vi "FPGAmacroTDC.vi"() -> ()   [LabVIEW 2017]
uses:
  <vilib>/Platform/TimedLoop/XDataNode/timing_clust.ctl
  <vilib>/Platform/TimedLoop/XDataNode/nitl_modes.ctl
  <vilib>/Platform/TimedLoop/XDataNode/wakeup.ctl
  <vilib>/rvi/Emulation/niFpgaGetClockAttributes.vi
  <vilib>/rvi/Emulation/niFpgaSctlEmulationGetInTimedLoop.vi
  <vilib>/rvi/Emulation/niFpgaEmulationReportErrorSimple.vi
  <vilib>/rvi/Emulation/niFpgaProcessEmulError.vi
  <vilib>/rvi/eio/common/nirviEmuTemplateMethod_errors.vi
  <vilib>/rvi/Emulation/niFpgaCriticalErrorInLSC.vi
  <vilib>/rvi/Memory/Memory_Emulation/nirvimemoryEmulation.vi
  <vilib>/rvi/Memory/Memory_Emulation/nirvimemoryFastEmulation.vi
  <vilib>/rvi/DataTransferAndStorage/Container/Common/niFpgaContainerGetUniqueNameForEmu.vi
  <vilib>/rvi/Memory/Memory_Emulation/niFpgaMemoryEmulationCacheClearOnFirstRun.vi
  <vilib>/rvi/Memory/Memory_Emulation/nirvimemoryEmulationManagerCache_MakeExclusive.vi
  <vilib>/rvi/Memory/Memory_Emulation/niFpgaMemoryEmulationValidateCache.vi
  <vilib>/rvi/Memory/Memory_Emulation/nirvimemoryEmulationManagerCache_InsertValue.vi
  <vilib>/Utility/error.llb/Clear Errors.vi
  <vilib>/rvi/Memory/Memory_Emulation/nirvimemoryEmulationManagerCache_ReleaseExclusive.vi
  <vilib>/rvi/Memory/Memory_Emulation/nirvimemoryEmulationManagerCache_GetValue.vi
  <vilib>/rvi/Emulation/niFpgaEmulationIsFPGAContextNoSignature.vi
  <vilib>/rvi/Memory/Memory_Emulation/nirvimemoryEmulationManagerCache_SetValue.vi
  <vilib>/rvi/Emulation/niFpgaSctlEmulationResourceMgr.vi
  <vilib>/rvi/DataTransferAndStorage/Container/Common/niFpgaContainerExecOnDevCompGetState.vi
  <vilib>/rvi/errors/niFpgaSetErrorForExecOnDevCompSimple.vi
  <vilib>/rvi/eio/common/nirviEmuReportErrorAndStop.vi
  <vilib>/rvi/FIFO/Fifo_Resource/nirvififoEmulationSetSize.vi
  <vilib>/rvi/FIFO/Fifo_Resource/nirviFifoEmulationQueueMgr.vi
  <instcachedir>/0/nirviFifoEmulationQueueMgr_E5CAEC123FF24DC58D834DCA3CDAA9B5.lvgen/nirviFifoEmulationQueueMgr_E5CAEC123FF24DC58D834DCA3CDAA9B5_001.vi
  <vilib>/rvi/FIFO/Fifo_Resource/nirvififoEmulationDetermineInputValidOut.vi
  <vilib>/rvi/FIFO/Fifo_Resource/nirvififoEmulationCreateLock.vi
  <vilib>/rvi/FIFO/Fifo_Resource/nirvififoEmulationObtainLock.vi
  <vilib>/rvi/FIFO/Fifo_Resource/nirvififoEmulationReleaseLock.vi
  <vilib>/rvi/occurrence/nirviWaitOnOccurrenceBase.vi
  <vilib>/rvi/errors/nirviReportUnexpectedCaseInternalError.vi
  <vilib>/rvi/errors/nirviReportUnexpectedCaseInternalError (U32).vi
  <vilib>/rvi/interface/RandomDataEmulation/niFpgaRandomDataHandleErrors.vi
  <vilib>/rvi/DataTransferAndStorage/Container/Common/niFpgaContainerSetEmuInfo.vi
  <vilib>/eio/EIONode/EIONode.xnode
  <vilib>/Platform/TimedLoop/XDataNode/XDataNode.xnode
  <vilib>/rvi/DataTransferAndStorage/Container/XNode/niFpgaContainer.xnode
  <vilib>/rvi/FIFO/Fifo_Resource/niFpgaFifoEmulationRefIn.vi
  <vilib>/rvi/interface/RandomDataEmulation/nirviRandomDataFpgaReadWriteTemplate.vi
  <vilib>/addons/control/pid/fpga.llb/XNode/niFpgaPID.xnode
  <vilib>/rvi/LocalResourceManager/LocalResourceManager.xnode
  <vilib>/Platform/TimedLoop/XDataNode/XDNodeRunTimeDep.lvlib
panel:
  out "new data":bool=TRUE
  out "tau":u32
  in  "N photons":u32
  in  "Acquire times":bool
  in  "AO4 max":i16 min=0 max=3277
  in  "AO7":i16
  in  "AO6":i16
  in  "AO5":i16
  in  "D31":bool
  in  "D30":bool
  in  "D29":bool
  in  "D28":bool
  in  "D27":bool
  in  "D26":bool
  in  "D25":bool
  in  "D24":bool
  out "Seq DO bits":u64
  in  "High power":bool
  in  "Reinitialise controller":bool
  in  "PID gains":T1={"Proportional gain Kc"=0.0, "Integral time Ti [min]"=2.0, "Derivative time Td [min]"=0.0}
  in  "Controller output range":T2={"Output high"=10.0, "Output low"=-10.0}
  out "Control Signal 2":i16
  in  "Setpoint (L)":fxp<+/-,16,16> format="%.3f"
  out "Filtered Input":fxp<+/-,16,16>
  out "Filtered Input":i16(graph)
  out "Control Signal":i16(graph)
  out "Input Signal / mV":fxp<+/-,19,14> format="%.3g"
  out "Control Signal / mV":fxp<+/-,19,14> format="%.3g"
  in  "Setpoint (H)":fxp<+/-,16,16>
  in  "override noise eater?":bool
  in  "D23":bool
  in  "D22":bool
  in  "D21":bool
  in  "D20":bool
  in  "D19":bool
  in  "D18":bool
  in  "D17":bool
  in  "D16":bool
  in  "D15":bool
  in  "D14":bool
  in  "D13":bool
  in  "D12":bool
  out "coerced AO3 fl scan":i16
  in  "AO3 fl scan":i16
  out "Seq AO bits":u8
  in  "trigger data":u8
  in  "AO data":u8
  in  "time data":u32
  in  "count data":u8
  out "data waiting":bool
  in  "pulse number":u32
  in  "digout data":u64
  in  "Send photons?":bool
  out "Numeric":u32
  out "Array":u32[](array[numeric])
  in  "DIO11":bool
  in  "DIO5":bool
  in  "DIO4":bool
  in  "dds/ag":bool
  in  "AO1":bool
  in  "AO1 off":i16
  in  "AO1 on":i16
  in  "AO4":bool
  in  "AO4 off":i16
  in  "AO4 on":i16
  out "PMT COUNTS D":u32
  out "PMT COUNTS C":u32
  in  "AO3":bool
  in  "AO2":bool
  in  "AO3 off":i16
  in  "AO2 off":i16
  in  "AO3 on":i16
  in  "AO2 on":i16
  out "Error type":u8
  out "Error?":bool
  in  "Fl scan time":u32
  in  "Enum":enum16{"Pulse", "Fluorescence"}(ring)
  out "bin number":u32
  in  "ticks per bin":u32=40000000
  out "Frequency Chart":u32(graph)
  out "loop counter":u64
  in  "AOM":bool
  in  "DIO10":bool
  in  "Microwave":bool
  in  "EOM":bool
  in  "DIO6":bool
  in  "DIO7":bool
  in  "DIO9":bool
  in  "DIO8":bool
  out "PMT saturation":bool
  out "Slave loop selector":u8
  in  "AO7":i16
  in  "AO6":i16
  in  "start sequence":bool
  in  "Line trig?":bool
  in  "# of pulses":i32
  in  "Debug counts?":bool
  in  "# of runs":i32
  out "Fifo Timed Out (B)":bool
  out "PMT COUNTS A":u32
  out "Fifo Timed Out (A)":bool
  out "PMT COUNTS B":u32
  # "Seb AO"
  # "Scan type:"
  # "Load AO memory"
  # "Fluorescence scan"
  # "Pulse sequencer"
  # "Globals"
  # "369 drift lock"
  # "List of error types:\n\n1: AO3 (AOM) voltage out of range."
  # "Crud:"
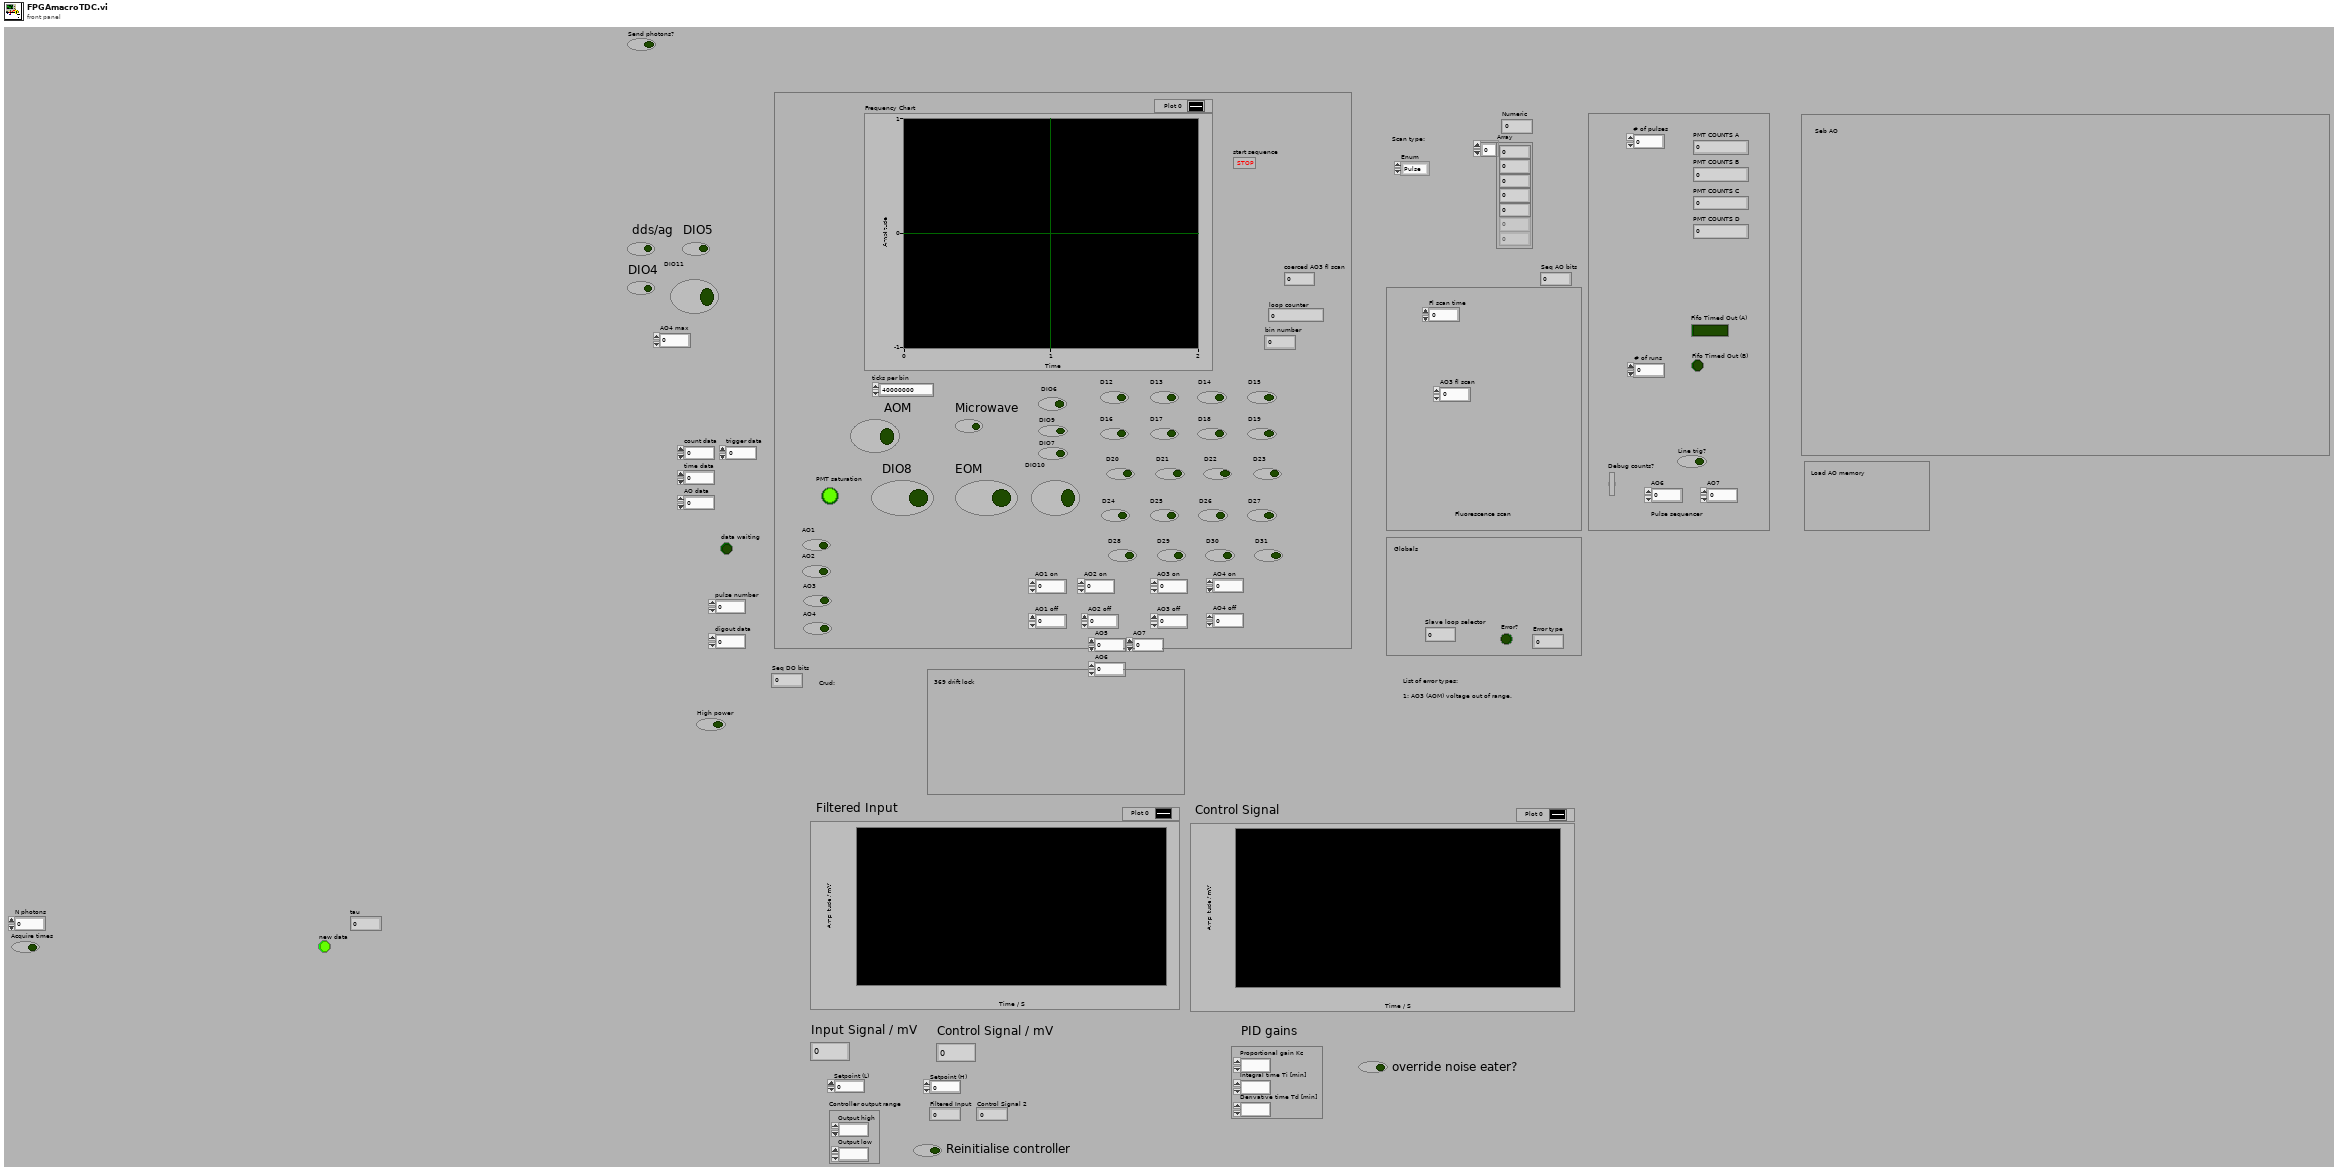
[diagram p1: front panel]
types:
  T1 = cluster{"Proportional gain Kc":fxp<+/-,16,8>, "Integral time Ti [min]":fxp<+/-,16,8>, "Derivative time Td [min]":fxp<+/-,16,8>}
  T2 = cluster{"Output high":fxp<+/-,16,16>, "Output low":fxp<+/-,16,16>}
  T3 = typedef "XDNodeRunTimeDep.lvlib/timing_clust.ctl" = cluster{"Expected End [f-1]":u64, "Actual End [f-1]":u64, "Finished Late? [f-1]":bool, "Expected End [i-1]":u64, "Actual End [i-1]":u64, "Finished Late? [i-1]":bool, "Expected Start [i]":u64, "Actual Start [i]":u64, "Expected Start [f]":u64, "Actual Start [f]":u64, "Source Name":string, "Structure Name":string, "Period":i64, "Deadline":i64, "Offset":i64, "Start":i64, "Priority":i32, "Timeout":i32, "Mode":T4, "Wakeup Reason":T5, "Error":errorcluster, "Source Type":string, "Secondary Source Type":string, "Global End Time":u64, "Global Start Time":u64, "Frame Duration":u64, "Iteration Duration":u64, "Assigned CPU":i32, "I/O Scan Engine Mode":u32}
  T4 = typedef "XDNodeRunTimeDep.lvlib/nitl_modes.ctl" = enum32{"No Change", "Process missed periods, maintain original phase", "Discard missed periods, maintain original phase", "Process missed periods, ignore original phase", "Discard missed periods, ignore original phase"}
  T5 = typedef "XDNodeRunTimeDep.lvlib/wakeup.ctl" = enum32{"Normal", "Aborted", "Asynchronous wakeup", "Timing source error", "Timed loop error", "Timeout"}
  T6 = cluster{"Boolean array[0]":bool, "Boolean array[1]":bool, "Boolean array[2]":bool, "Boolean array[3]":bool}
  T7 = cluster{"proportional gain (Kc)":i16, "integral gain (Kc*Ts/Ti)":i16, "derivative gain (Kc*Td/Ts)":i16}
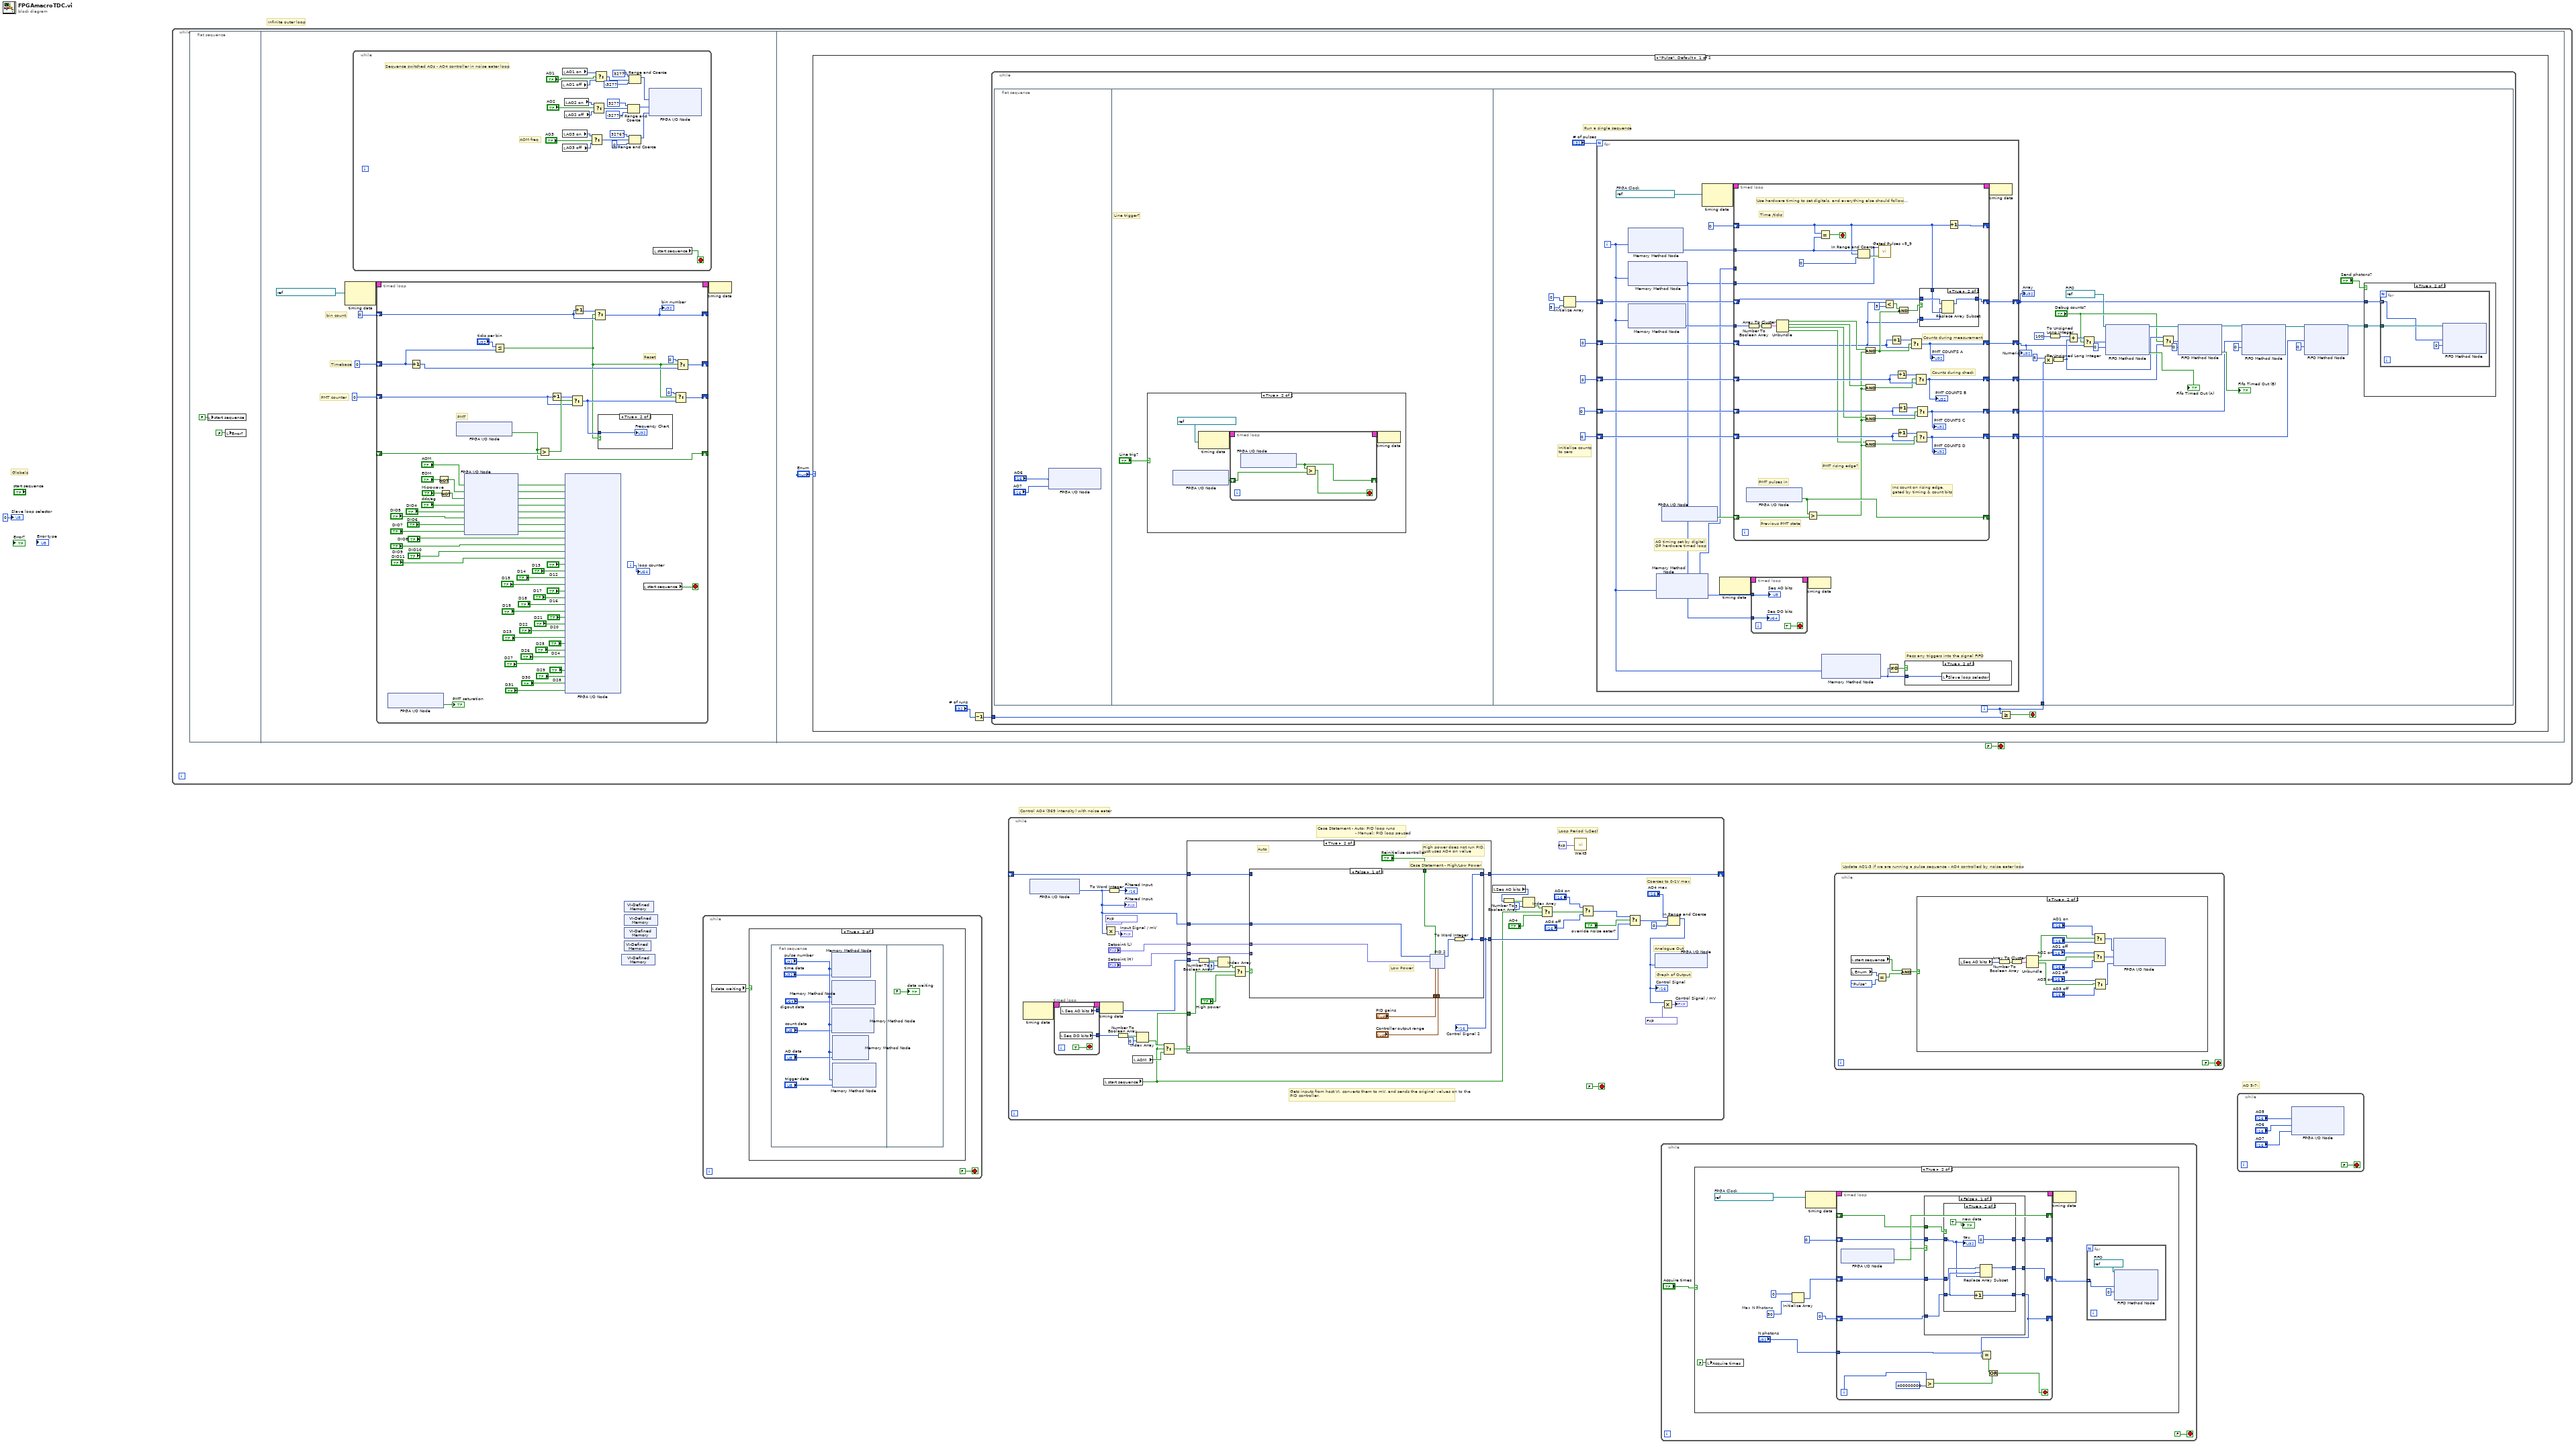
[diagram p0: block diagram]
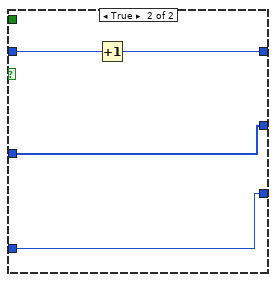
[diagram p4: hidden frame]
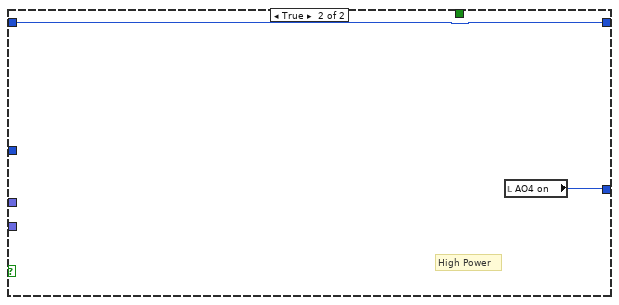
[diagram p6: hidden frame]
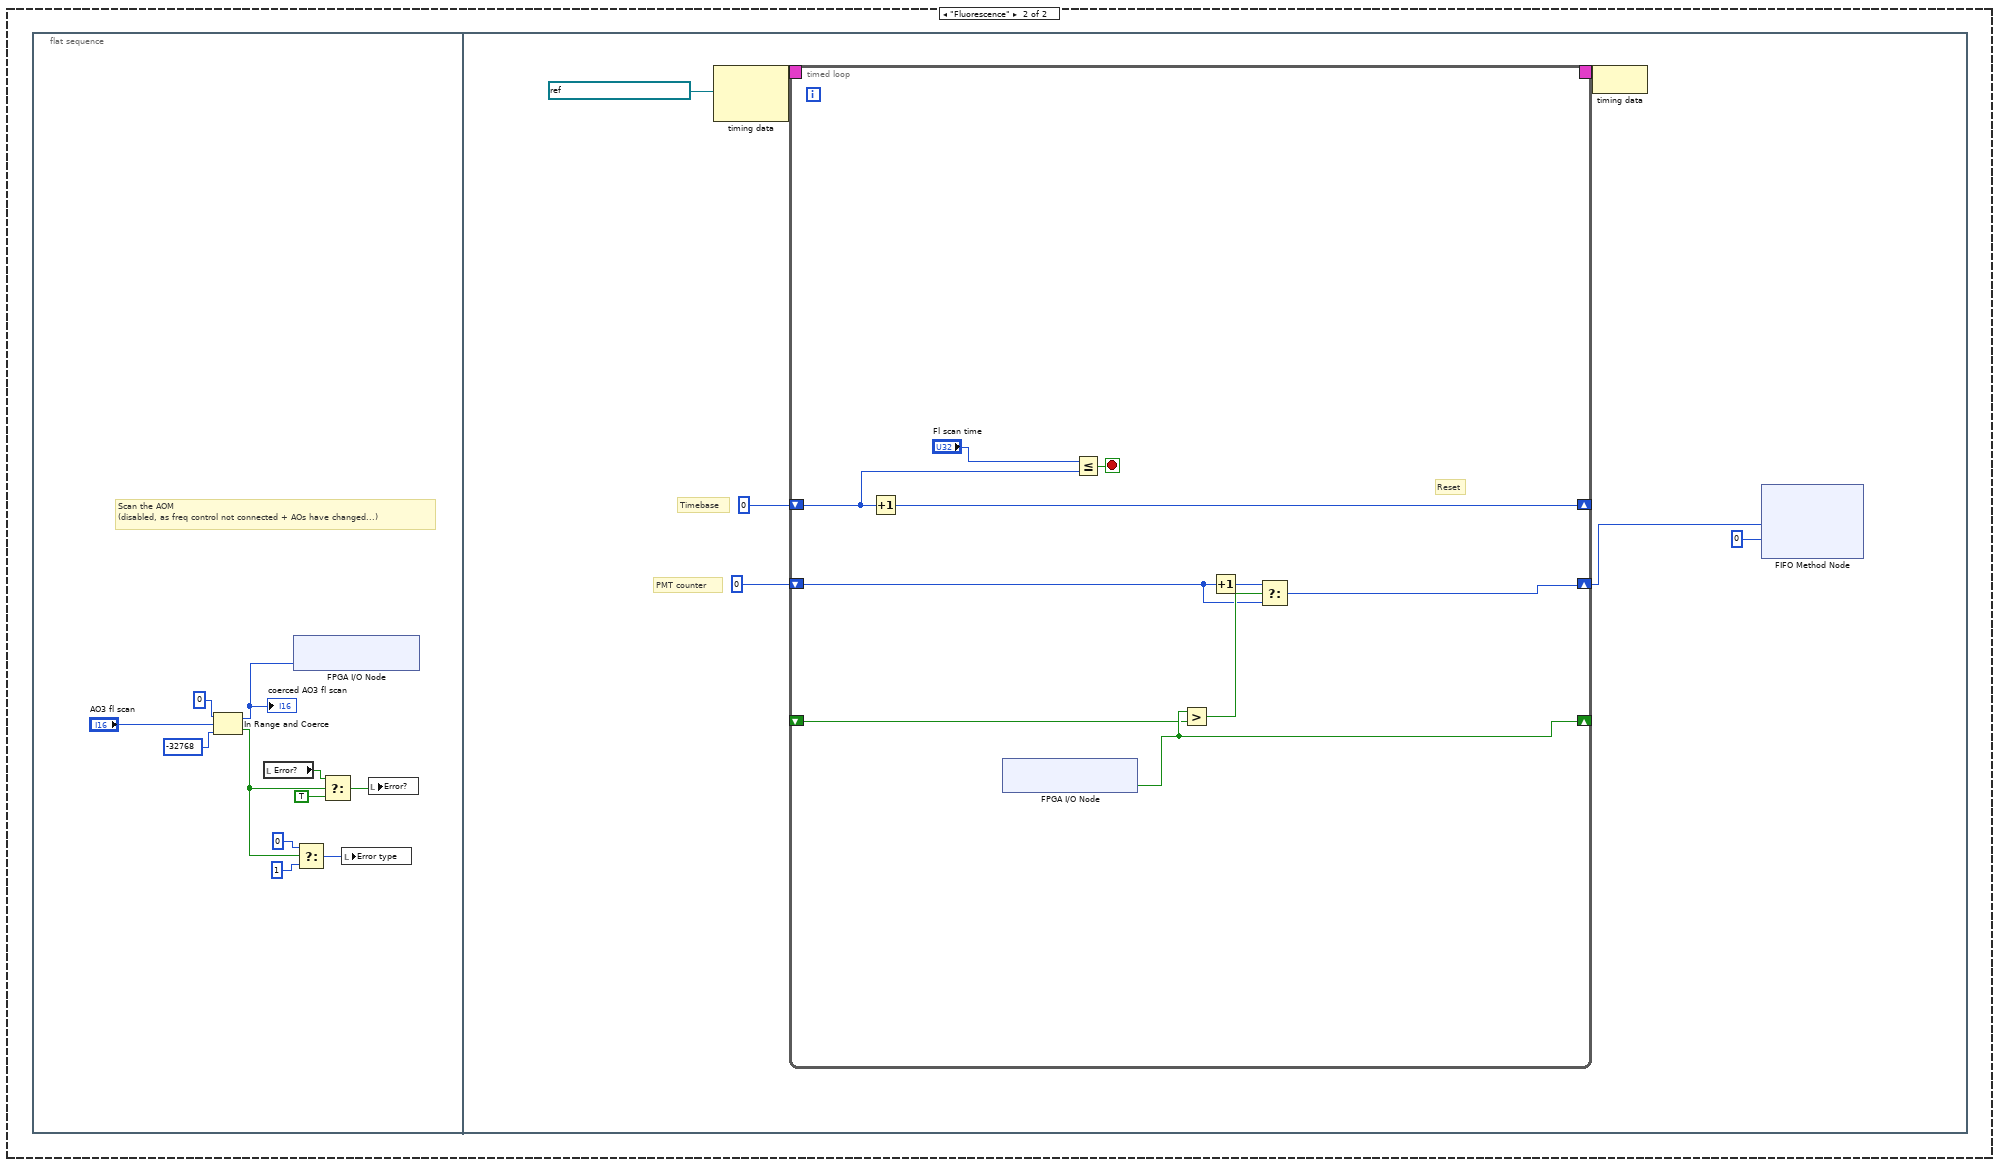
[diagram p14: hidden frame]
diagram:
  # "Control AO4 (369 intensity) with noise eater"
  # "Update AO1-3 if we are running a pulse sequence - AO4 controlled by noise eater loop"
  # "AO 5-7:"
  # "Globals"
  # "Infinite outer loop"
  n1 = while {
    stop <- FALSE stop-if-true
    n2 = flat-sequence {
      frame #0 {
        n3 = local write "start sequence"(FALSE ("start sequence")) -> ()
        n4 = local write "Error?"(FALSE ("Error?")) -> ()
      }
      frame #1 {
        # "bin count"
        # "PMT counter"
        # "Timebase"
        n5 = node-c288(refnum<k21> "40 MHz Onboard Clock" ("FPGA Clock To Enable")) -> (w10:T3)  [unwired: 1 in]
        n6 = while {
          stop <- w93 stop-if-true
          # "AOM freq"
          # "Sequence switched AOs - AO4 controller in noise eater loop"
          n7 = local read "AO1 off"() -> (w75:i16)
          n8 = local read "AO1 on"() -> (w76:i16)
          n9 = local read "AO3 on"() -> (w86:i16)
          n10 = local read "AO3 off"() -> (w85:i16)
          n11 = local read "AO2 on"() -> (w88:i16)
          n12 = local read "AO2 off"() -> (w87:i16)
          n13 = Select(t=w86, s="AO3", f=w85) -> (s? t:f=w82:i16)
          n14 = Select(t=w88, s="AO2", f=w87) -> (s? t:f=w81:i16)
          n15 = Select(t=w76, s="AO1", f=w75) -> (s? t:f=w77:i16)
          n16 = In Range and Coerce(upper limit=i16 3277, x=w81, lower limit=i16 -3277) -> (coerced(x)=w92:i16)  [unwired: 1 out]
          n17 = In Range and Coerce(upper limit=i16 32767, x=w82, lower limit=i16 0) -> (coerced(x)=w89:i16)  [unwired: 1 out]
          n18 = In Range and Coerce(upper limit=i16 3277, x=w77, lower limit=i16 -3277) -> (coerced(x)=w78:i16)  [unwired: 1 out]
          n19 = xnode "FPGA I/O Node"("Connector0/AO1"=w78, "Connector0/AO2"=w92, "Connector0/AO3"=w89) -> ()  [unwired: 3 in, 3 out]
          n20 = local read "start sequence"() -> (w93:bool)
        }
        n21 = timed-loop {
          timing: w10 -> [_]
          timing-out: [_] -> w9
          shift-right: [w62] -> _
          shift-left: u32 0 -> [w55]
          shift-right: [w60] -> _
          shift-left: u32 0 -> [w57]
          shift-right: [w45] -> _
          shift-left: _ -> [w53]
          shift-right: [w49] -> _
          shift-left: u32 0 -> [w47]
          i -> [w54]
          stop <- w50 stop-if-true
          # "PMT"
          # "Reset"
          n22 = xnode "FPGA I/O Node"() -> ("Connector0/DIO13"=→"PMT saturation":bool)  [unwired: 1 in, 1 out]
          n23 = Increment(x=w55) -> (x+1=w64:u32)
          n24 = Not(x="EOM") -> (.not. x?=w12:bool)
          n25 = Not(x="Microwave") -> (.not. x?=w43:bool)
          n26 = xnode "FPGA I/O Node"() -> ("Connector0/DIO15"=w45:bool)  [unwired: 1 in, 1 out]
          n27 = xnode "FPGA I/O Node"("Connector0/DIO0"="AOM", "Connector0/DIO1"=w12, "Connector0/DIO2"=w43, "Connector0/DIO3"="dds/ag", "Connector0/DIO4"="DIO4", "Connector0/DIO5"="DIO5", "Connector0/DIO6"="DIO6", "Connector0/DIO7"="DIO7") -> ()  [unwired: 8 in, 8 out]
          n28 = Less Or Equal?(x="ticks per bin", y=w55) -> (x <= y?=w46:bool)
          n29 = Greater?(x=w45, y=w53) -> (0:w58:bool)
          n30 = Increment(x=w57) -> (x+1=w61:u32)
          n31 = xnode "FPGA I/O Node"("Connector1/DIO0"="AOM", "Connector1/DIO1"=w12, "Connector1/DIO2"=w43, "Connector1/DIO3"="dds/ag", "Connector1/DIO4"="DIO4", "Connector1/DIO5"="DIO5", "Connector1/DIO6"="DIO6", "Connector1/DIO7"="DIO7", "Connector1/DIO8"="DIO8", "Connector1/DIO9"="DIO9", "Connector1/DIO10"="DIO10", "Connector1/DIO11"="DIO11", "Connector1/DIO12"="D12", "Connector1/DIO13"="D13", "Connector1/DIO14"="D14", "Connector1/DIO15"="D15", "Connector1/DIO16"="D16", "Connector1/DIO17"="D17", "Connector1/DIO18"="D18", "Connector1/DIO19"="D19", "Connector1/DIO20"="D20", "Connector1/DIO21"="D21", "Connector1/DIO22"="D22", "Connector1/DIO23"="D23", "Connector1/DIO24"="D24", "Connector1/DIO25"="D25", "Connector1/DIO26"="D26", "Connector1/DIO27"="D27", "Connector1/DIO28"="D28", "Connector1/DIO29"="D29", "Connector1/DIO30"="D30", "Connector1/DIO31"="D31") -> ()  [unwired: 32 in, 32 out]
          n32 = Select(t=w61, s=w58, f=w57) -> (s? t:f=w51:u32)
          n33 = Increment(x=w47) -> (x+1=w48:u32)
          n34 = Select(t=w48, s=w46, f=w47) -> (s? t:f=w49:u32)
          "bin number" <- w49
          n35 = case shown="True" w46 {
            tunnel: w51 -> [_ w65]
            frame False {
            }
            frame True {
              "Frequency Chart" <- w65
            }
          }
          n36 = local read "start sequence"() -> (w50:bool)
          n37 = Select(t=u32 0, s=w46, f=w51) -> (s? t:f=w60:u32)
          n38 = Select(t=u32 0, s=w46, f=w64) -> (s? t:f=w62:u32)
          "loop counter" <- w54
        }
        n39 = node-c288(w9) -> ()
      }
      frame #2 {
        n40 = case shown="\"Pulse\", Default" "Enum" {
          frame "Pulse", Default {
            n41 = Decrement(x="# of runs") -> (x-1=w95:i32)
            n42 = while {
              tunnel: w95 -> [w98]
              i -> [w99]
              stop <- w97 stop-if-true
              n43 = flat-sequence {
                tunnel: w99 -> [w131]
                frame #0 {
                  n44 = xnode "FPGA I/O Node"("Connector0/AO6"="AO6", "Connector0/AO7"="AO7") -> ()  [unwired: 2 in, 2 out]
                }
                frame #1 {
                  # "Line trigger?"
                  n45 = case shown="True" "Line trig?" {
                    frame False {
                    }
                    frame True {
                      n46 = xnode "FPGA I/O Node"() -> ("Connector0/DIO14"=w103:bool)  [unwired: 1 in, 1 out]
                      n47 = node-c288(refnum<k21> "40 MHz Onboard Clock" ("Source Name")) -> (w106:T3)
                      n48 = timed-loop {
                        timing: w106 -> [_]
                        timing-out: [_] -> w105
                        shift-right: [w108] -> _
                        shift-left: w103 -> [w109]
                        stop <- w107 stop-if-true
                        n49 = xnode "FPGA I/O Node"() -> ("Connector0/DIO14"=w108:bool)  [unwired: 1 in, 1 out]
                        n50 = Greater?(x=w108, y=w109) -> (0:w107:bool)
                      }
                      n51 = node-c288(w105) -> ()
                    }
                  }
                }
                frame #2 {
                  w119 = refnum<k21> "U32 FIFO"  # FIFO
                  # "Run a single sequence"
                  # "Initialize counts\nto zero"
                  n52 = Initialize Array(u32 0 ("element"), 5 ("dimension size")) -> (w120:u32[])
                  n53 = for {
                    N: "# of pulses" -> [_]
                    shift-right: [w176] -> w137
                    shift-left: u32 0 -> [w174]
                    shift-right: [w175] -> w139
                    shift-left: u32 0 -> [w173]
                    shift-right: [w168] -> w124
                    shift-left: u32 0 -> [w169]
                    shift-right: [w166] -> w123
                    shift-left: u32 0 -> [w167]
                    shift-right: [w164] -> w116
                    shift-left: w120 -> [w165]
                    i -> [w161]
                    w177 = refnum<k21> "40 MHz Onboard Clock"  # FPGA Clock
                    # "AO timing set by digital\nOP hardware timed loop"
                    # "Pass any triggers into the signal FIFO"
                    n54 = xnode ("Memory Method Node")("Address"=w161) -> ("Data"=w158:u64)  [unwired: 1 in, 1 out]
                    n55 = xnode ("Memory Method Node")("Address"=w161) -> ("Data"=w163:u32)  [unwired: 1 in, 1 out]
                    n56 = xnode ("Memory Method Node")("Address"=w161) -> ("Data"=w162:u8)  [unwired: 1 in, 1 out]
                    n57 = xnode ("Memory Method Node")("Address"=w161) -> ("Data"=w160:u8)  [unwired: 1 in, 1 out]
                    n58 = xnode "FPGA I/O Node"() -> ("Connector0/DIO15"=w171:bool)  [unwired: 1 in, 1 out]
                    n59 = node-c288(w177) -> (w179:T3)  [unwired: 1 in]
                    n60 = node-c288() -> (w157:T3)  [unwired: 1 in]
                    n61 = timed-loop {
                      timing: w179 -> [_]
                      timing-out: [_] -> w178
                      shift-right: [w219] -> w176
                      shift-left: w174 -> [w189]
                      shift-right: [w225] -> _
                      shift-left: w171 -> [w224]
                      shift-right: [w209] -> _
                      shift-left: u32 0 -> [w188]
                      shift-right: [w217] -> w175
                      shift-left: w173 -> [w221]
                      tunnel: w158 -> [w211]
                      tunnel: w162 -> [w210]
                      tunnel: w163 -> [w208]
                      shift-right: [w202] -> w168
                      shift-left: w169 -> [w204]
                      shift-right: [w198] -> w166
                      shift-left: w167 -> [w199]
                      shift-right: [w190] -> w164
                      shift-left: w165 -> [w192]
                      tunnel: w160 -> [_]
                      stop <- w218 stop-if-true
                      # "Use hardware timing to set digitals, and everything else should follow..."
                      # "Previous PMT state"
                      # "Counts during check"
                      # "Counts during measurement"
                      # "Time /ticks"
                      # "Inc count on rising edge,\ngated by timing & count bits"
                      # "PMT rising edge?"
                      # "PMT pulses in"
                      n62 = xnode "FPGA I/O Node"() -> ("Connector0/DIO15"=w225:bool)  [unwired: 1 in, 1 out]
                      n63 = Number To Boolean Array(number=w210) -> (Boolean array=w214:bool[])
                      n64 = Array To Cluster(array=w214) -> (cluster=w213:T6)
                      n65 = Unbundle(w213) -> ("Boolean array[0]"=w207:bool, "Boolean array[1]"=w212:bool, "Boolean array[2]"=w203:bool, "Boolean array[3]"=w196:bool)
                      n66 = Greater?(x=w225, y=w224) -> (0:w197:bool)
                      n67 = Equal?(x=w188, y=w208) -> (x = y?=w218:bool)
                      n68 = In Range and Coerce(upper limit=w208, x=w188, lower limit=u32 0) -> (In Range?=w216:bool)  [unwired: 1 out]
                      n69 = And(x=w207, y=w197) -> (x .and. y?=w193:bool)
                      n70 = And(x=w212, y=w197) -> (x .and. y?=w220:bool)
                      n71 = And(x=w203, y=w197) -> (x .and. y?=w205:bool)
                      n72 = And(x=w196, y=w197) -> (x .and. y?=w200:bool)
                      n73 = call "Gated Pulses v5_9.vi"("Gate"=w216, "Pulse bits"=w211) -> ()  [unwired: 3 in]
                      n74 = Less?(x=w189, y=i16 5) -> (x < y?=w194:bool)
                      n75 = Increment(x=w189) -> (x+1=w223:u32)
                      n76 = Increment(x=w221) -> (x+1=w222:u32)
                      n77 = Increment(x=w199) -> (x+1=w201:u32)
                      n78 = Increment(x=w204) -> (x+1=w206:u32)
                      n79 = And(x=w194, y=w193) -> (x .and. y?=w191:bool)
                      n80 = Select(t=w223, s=w193, f=w189) -> (s? t:f=w219:u32)
                      "PMT COUNTS A" <- w219
                      n81 = Select(t=w222, s=w220, f=w221) -> (s? t:f=w217:u32)
                      "PMT COUNTS B" <- w217
                      n82 = Select(t=w201, s=w200, f=w199) -> (s? t:f=w198:u32)
                      "PMT COUNTS D" <- w198
                      n83 = Select(t=w206, s=w205, f=w204) -> (s? t:f=w202:u32)
                      "PMT COUNTS C" <- w202
                      n84 = case shown="True" w191 {
                        tunnel: w192 -> [w226 w230]
                        tunnel: [w226 w229] -> w190
                        tunnel: w189 -> [_ w227]
                        tunnel: w188 -> [_ w228]
                        frame False {
                        }
                        frame True {
                          n85 = Replace Array Subset(array=w230, new element=w228, index=w227) -> (w229:u32[])
                        }
                      }
                      n86 = Increment(x=w188) -> (x+1=w209:u32)
                    }
                    n87 = timed-loop {
                      timing: w157 -> [_]
                      timing-out: [_] -> w156
                      tunnel: w160 -> [w182]
                      tunnel: w158 -> [w181]
                      stop <- TRUE stop-if-true
                      "Seq AO bits" <- w182
                      "Seq DO bits" <- w181
                    }
                    n88 = node-c288(w156) -> ()
                    n89 = xnode ("Memory Method Node")("Address"=w161) -> ("Data"=w159:u8)  [unwired: 1 in, 1 out]
                    n90 = Not Equal To 0?(x=w159) -> (x != 0?=w170:bool)
                    n91 = case shown="True" w170 {
                      tunnel: w159 -> [_ w187]
                      frame False {
                      }
                      frame True {
                        n92 = local write "Slave loop selector"(w187) -> ()
                      }
                    }
                    n93 = node-c288(w178) -> ()
                  }
                  "Array" <- w116
                  "Numeric" <- w137
                  n94 = Multiply(x=5 ("y"), y=w131) -> (x*y=w144:i32)
                  n95 = To Unsigned Long Integer(number=i16 100) -> (unsigned 32bit integer=w145:u32)
                  n96 = To Unsigned Long Integer(number=w144) -> (unsigned 32bit integer=w143:u32)
                  n97 = Add(x=w145, y=w143) -> (x+y=w141:u32)
                  n98 = Select(t=w141, s="Debug counts?", f=w137) -> (s? t:f=w140:u32)
                  n99 = xnode ("FIFO Method Node")("Element"=w140, "Timeout"=0, "FIFO In"=w119) -> ("Timed Out?"=→"Fifo Timed Out (A)":bool, "FIFO Out"=w148:refnum<k21>)
                  n100 = Select(t=w143, s="Debug counts?", f=w139) -> (s? t:f=w142:u32)
                  n101 = xnode ("FIFO Method Node")("Element"=w142, "Timeout"=0, "FIFO In"=w148) -> ("Timed Out?"=→"Fifo Timed Out (B)":bool, "FIFO Out"=w128:refnum<k21>)
                  n102 = xnode ("FIFO Method Node")("Element"=w124, "Timeout"=0, "FIFO In"=w128) -> ("FIFO Out"=w127:refnum<k21>)  [unwired: 1 out]
                  n103 = xnode ("FIFO Method Node")("Element"=w123, "Timeout"=0, "FIFO In"=w127) -> ("FIFO Out"=w117:refnum<k21>)  [unwired: 1 out]
                  n104 = case shown="True" "Send photons?" {
                    tunnel: w117 -> [_ w152]
                    tunnel: w116 -> [_ w151]
                    frame False {
                    }
                    frame True {
                      n105 = for {
                        tunnel: w152 -> [w155]
                        tunnel: w151 -> [w153] mode=indexing
                        n106 = xnode ("FIFO Method Node")("Element"=w153, "Timeout"=0, "FIFO In"=w155) -> ()  [unwired: 2 out]
                      }
                    }
                  }
                }
              }
              n107 = Greater Or Equal?(x=w99, y=w98) -> (x >= y?=w97:bool)
            }
          }
          frame "Fluorescence" {
            n108 = flat-sequence {
              frame #0 {
                # "Scan the AOM\n(disabled, as freq control not connected + AOs have changed...)"
                n109 = In Range and Coerce(upper limit=i16 0, x="AO3 fl scan", lower limit=i16 -32768) -> (coerced(x)=w245:i16, In Range?=w240:bool)
                "coerced AO3 fl scan" <- w245
                n110 = local read "Error?"() -> (w244:bool)
                n111 = xnode "FPGA I/O Node"("Connector0/AO3"=w245) -> ()  [unwired: 1 in, 1 out]
                n112 = Select(t=u8 0, s=w240, f=u8 1) -> (s? t:f=w241:u8)
                n113 = Select(t=w244, s=w240, f=TRUE) -> (s? t:f=w242:bool)
                n114 = local write "Error type"(w241) -> ()
                n115 = local write "Error?"(w242) -> ()
              }
              frame #1 {
                # "PMT counter"
                # "Timebase"
                n116 = node-c288(refnum<k21> "40 MHz Onboard Clock" ("FPGA Clock To Enable")) -> (w254:T3)  [unwired: 1 in]
                n117 = timed-loop {
                  timing: w254 -> [_]
                  timing-out: [_] -> w253
                  shift-right: [w255] -> _
                  shift-left: u32 0 -> [w261]
                  shift-right: [w257] -> w248
                  shift-left: u32 0 -> [w262]
                  shift-right: [w260] -> _
                  shift-left: _ -> [w259]
                  stop <- w256 stop-if-true
                  # "Reset"
                  n118 = Increment(x=w261) -> (x+1=w255:u32)
                  n119 = xnode "FPGA I/O Node"() -> ("Connector0/DIO15"=w260:bool)  [unwired: 1 in, 1 out]
                  n120 = Less Or Equal?(x="Fl scan time", y=w261) -> (x <= y?=w256:bool)
                  n121 = Greater?(x=w260, y=w259) -> (0:w263:bool)
                  n122 = Increment(x=w262) -> (x+1=w264:u32)
                  n123 = Select(t=w264, s=w263, f=w262) -> (s? t:f=w257:u32)
                }
                n124 = node-c288(w253) -> ()
                n125 = xnode ("FIFO Method Node")("Element"=w248, "Timeout"=0) -> ()  [unwired: 1 in, 2 out]
              }
            }
          }
        }
      }
    }
  }
  n126 = xnode "VI-Defined Memory"() -> ()  [unwired: 1 out]
  n127 = xnode "VI-Defined Memory"() -> ()  [unwired: 1 out]
  n128 = xnode "VI-Defined Memory"() -> ()  [unwired: 1 out]
  n129 = xnode "VI-Defined Memory"() -> ()  [unwired: 1 out]
  n130 = xnode "VI-Defined Memory"() -> ()  [unwired: 1 out]
  n131 = while {
    stop <- FALSE stop-if-true
    n132 = local read "data waiting"() -> (w272:bool)
    n133 = case shown="True" w272 {
      frame False {
      }
      frame True {
        n134 = flat-sequence {
          frame #0 {
            n135 = xnode ("Memory Method Node")("Address"="pulse number", "Data"="time data") -> ()  [unwired: 1 in, 1 out]
            n136 = xnode ("Memory Method Node")("Address"="pulse number", "Data"="digout data") -> ()  [unwired: 1 in, 1 out]
            n137 = xnode ("Memory Method Node")("Address"="pulse number", "Data"="count data") -> ()  [unwired: 1 in, 1 out]
            n138 = xnode ("Memory Method Node")("Address"="pulse number", "Data"="AO data") -> ()  [unwired: 1 in, 1 out]
            n139 = xnode ("Memory Method Node")("Address"="pulse number", "Data"="trigger data") -> ()  [unwired: 1 in, 1 out]
          }
          frame #1 {
            "data waiting" <- FALSE
          }
        }
      }
    }
  }
  n140 = while {
    shift-right: [w292] -> _
    shift-left: _ -> [w291]
    stop <- FALSE stop-if-true
    # "Coerces to 0-1V max"
    # "Graph of Output"
    # "Gets inputs from host VI, converts them to mV, and sends the original values on to the PID controller."
    # "Case Statement - Auto: PID loop runs\n                            - Manual: PID loop paused"
    # "Analogue Out"
    # "Loop Period (uSec)"
    n141 = node-c288() -> (w294:T3)  [unwired: 1 in]
    n142 = xnode "FPGA I/O Node"() -> ("Connector0/AI0"=w280:i16)  [unwired: 1 in, 1 out]
    "Filtered Input" <- w280
    n143 = timed-loop {
      timing: w294 -> [_]
      timing-out: [_] -> w293
      tunnel: [w319] -> w306
      tunnel: [w318] -> w295
      stop <- TRUE stop-if-true
      n144 = local read "Seq DO bits"() -> (w319:u64)
      n145 = local read "Seq AO bits"() -> (w318:u8)
    }
    n146 = node-c288(w293) -> ()
    n147 = local read "start sequence"() -> (w296:bool)
    n148 = Multiply(x=fxp<+,10,-1> 0.30517578125, y=w280) -> (x*y=→"Input Signal / mV":fxp<+/-,26,15>)
    n149 = To Word Integer(number=w280) -> (16bit integer=→"Filtered Input":i16)
    n150 = Number To Boolean Array(number=w306) -> (Boolean array=w308:bool[])
    n151 = local read "AOM"() -> (w305:bool)
    n152 = Index Array(array=w308, index=0) -> (element=w303:bool)
    n153 = Select(t=w303, s=w296, f=w305) -> (s? t:f=w304:bool)
    n154 = case shown="True" w304 {
      tunnel: [w324 w329] -> w309
      tunnel: "Setpoint (L)" -> [_ w337]
      tunnel: "Setpoint (H)" -> [_ w336]
      tunnel: w296 -> [_ w335]
      tunnel: w295 -> [_ w328]
      tunnel: [w324 w327] -> w292
      tunnel: w291 -> [w324 w326]
      tunnel: w280 -> [_ w325]
      frame False {
        # "Manual"
      }
      frame True {
        # "High power does not run PID,\njust uses AO4 on value"
        # "Case Statement - High/Low Power"
        # "Auto"
        n155 = Number To Boolean Array(number=w328) -> (Boolean array=w331:bool[])
        n156 = Index Array(array=w331, index=3) -> (element=w330:bool)
        n157 = Select(t=w330, s=w335, f="High power") -> (s? t:f=w334:bool)
        n158 = case shown="False" w334 {
          tunnel: "Reinitialise controller" -> [w345 _]
          tunnel: "PID gains" -> [w347 _]
          tunnel: "Controller output range" -> [w346 _]
          tunnel: [w342 w377] -> w329
          tunnel: w337 -> [w344 _]
          tunnel: w336 -> [_ _]
          tunnel: [w342 w376] -> w327
          tunnel: w326 -> [_ w376]
          tunnel: w325 -> [w341 _]
          frame False {
            # "Low Power"
            n159 = xnode ("PID 2")("process variable"=w341, "reset?"=w345, "setpoint"=w344, "PID gains"=w347, "output range"=w346) -> ("output"=w343:i16)
            n160 = To Word Integer(number=w343) -> (16bit integer=w342:i16)
          }
          frame True {
            # "High Power"
            n161 = local read "AO4 on"() -> (w377:i16)
          }
        }
        "Control Signal 2" <- w329
      }
    }
    n162 = local read "Seq AO bits"() -> (w300:u8)
    n163 = Number To Boolean Array(number=w300) -> (Boolean array=w301:bool[])
    n164 = Index Array(array=w301, index=3) -> (element=w297:bool)
    n165 = Select(t=w297, s=w296, f="AO4") -> (s? t:f=w298:bool)
    n166 = call "Wait3"("Count(uSec)"=fxp<+,1,4> 8.0) -> ()  [unwired: 1 out]
    n167 = Select(t="AO4 on", s=w298, f="AO4 off") -> (s? t:f=w299:i16)
    n168 = Select(t=w299, s="override noise eater?", f=w309) -> (s? t:f=w287:i16)
    n169 = In Range and Coerce(upper limit="AO4 max", x=w287, lower limit=i16 0) -> (coerced(x)=w286:i16)  [unwired: 1 out]
    "Control Signal" <- w286
    n170 = xnode "FPGA I/O Node"("Connector0/AO4"=w286) -> ()  [unwired: 1 in, 1 out]
    n171 = Multiply(x=w286, y=fxp<+,10,-1> 0.30517578125) -> (x*y=→"Control Signal / mV":fxp<+/-,26,15>)
  }
  n172 = while {
    stop <- FALSE stop-if-true
    n173 = case shown="True" "Acquire times" {
      frame False {
      }
      frame True {
        w380 = u32 50  # Max N Photons
        w387 = refnum<k21> "40 MHz Onboard Clock"  # FPGA Clock
        n174 = local write "Acquire times"(FALSE ("Acquire times")) -> ()
        n175 = Initialize Array(u32 0, w380) -> (w383:u32[])
        n176 = node-c288(w387) -> (w390:T3)
        n177 = timed-loop {
          timing: w390 -> [_]
          timing-out: [_] -> w389
          shift-right: [w406] -> _
          shift-left: u32 0 -> [w407]
          shift-right: [w405] -> _
          shift-left: _ -> [w404]
          shift-right: [w403] -> w388
          shift-left: w383 -> [w402]
          tunnel: "N photons" -> [w401]
          shift-right: [w399] -> _
          shift-left: u32 0 -> [w400]
          i -> [w397]
          stop <- w394 stop-if-true
          n178 = xnode "FPGA I/O Node"() -> ("Connector0/DIO5"=w405:bool)  [unwired: 1 in, 1 out]
          n179 = Greater?(x=w397, y=400000000) -> (0:w396:bool)
          n180 = case shown="False" w405 {
            tunnel: w407 -> [w413 w428]
            tunnel: [w412 w427] -> w406
            tunnel: w404 -> [w414 _]
            tunnel: w402 -> [w411 w426]
            tunnel: [w410 w426] -> w403
            tunnel: w400 -> [w409 w425]
            tunnel: [w408 w425] -> w399
            frame False {
              n181 = case shown="True" w414 {
                tunnel: w413 -> [w417 w419]
                tunnel: [w417 i16 0] -> w412
                tunnel: w411 -> [w416 w421]
                tunnel: [w416 w418] -> w410
                tunnel: w409 -> [w415 w420]
                tunnel: [w415 w422] -> w408
                frame False {
                }
                frame True {
                  n182 = Increment(x=w420) -> (x+1=w422:u32)
                  n183 = Replace Array Subset(array=w421, new element=w419, index=w420) -> (w418:u32[])
                  "new data" <- TRUE ("new data")
                  "tau" <- w419
                }
              }
            }
            frame True {
              n184 = Increment(x=w428) -> (x+1=w427:u32)
            }
          }
          n185 = Equal?(x=w401, y=w399) -> (x = y?=w395:bool)
          n186 = Or(x=w395, y=w396) -> (x .or. y?=w394:bool)
        }
        n187 = node-c288(w389) -> ()
        n188 = for {
          tunnel: w388 -> [w392] mode=indexing
          w393 = refnum<k21> "U32 FIFO"  # FIFO
          n189 = xnode ("FIFO Method Node")("Element"=w392, "Timeout"=0, "FIFO In"=w393) -> ()  [unwired: 2 out]
        }
      }
    }
  }
  n190 = while {
    stop <- FALSE stop-if-true
    n191 = local read "start sequence"() -> (w437:bool)
    n192 = local read "Enum"() -> (w439:enum16{"Pulse", "Fluorescence"})
    n193 = Equal?(x=w439, y=enum16{"Pulse", "Fluorescence"}."Pulse" ("Enum")) -> (x = y?=w438:bool)
    n194 = And(x=w437, y=w438) -> (x .and. y?=w436:bool)
    n195 = case shown="True" w436 {
      frame False {
      }
      frame True {
        n196 = local read "Seq AO bits"() -> (w443:u8)
        n197 = Number To Boolean Array(number=w443) -> (Boolean array=w444:bool[])
        n198 = Array To Cluster(array=w444) -> (cluster=w445:T6)
        n199 = Unbundle(w445) -> ("Boolean array[0]"=w441:bool, "Boolean array[1]"=w442:bool, "Boolean array[2]"=w455:bool)  [unwired: 1 out]
        n200 = Select(t="AO2 on", s=w442, f="AO2 off") -> (s? t:f=w446:i16)
        n201 = Select(t="AO1 on", s=w441, f="AO1 off") -> (s? t:f=w452:i16)
        n202 = Select(t="AO3 on", s=w455, f="AO3 off") -> (s? t:f=w447:i16)
        n203 = xnode "FPGA I/O Node"("Connector0/AO1"=w452, "Connector0/AO2"=w446, "Connector0/AO3"=w447) -> ()  [unwired: 3 in, 3 out]
      }
    }
  }
  n204 = while {
    stop <- FALSE stop-if-true
    n205 = xnode "FPGA I/O Node"("Connector0/AO5"="AO5", "Connector0/AO6"="AO6", "Connector0/AO7"="AO7") -> ()  [unwired: 3 in, 3 out]
  }
  "Slave loop selector" <- u8 0 ("Slave loop selector")
